vi "OutputWrapper.vi"(0 "VI in":refnum<vi>, 1 "pass":bool, 2 "FinalCluster":T1) -> (3 "PASS":bool, 4 "error out":errorcluster, 5 "ats json out":string, 6 "formatted test json out":string)   [LabVIEW 2019]
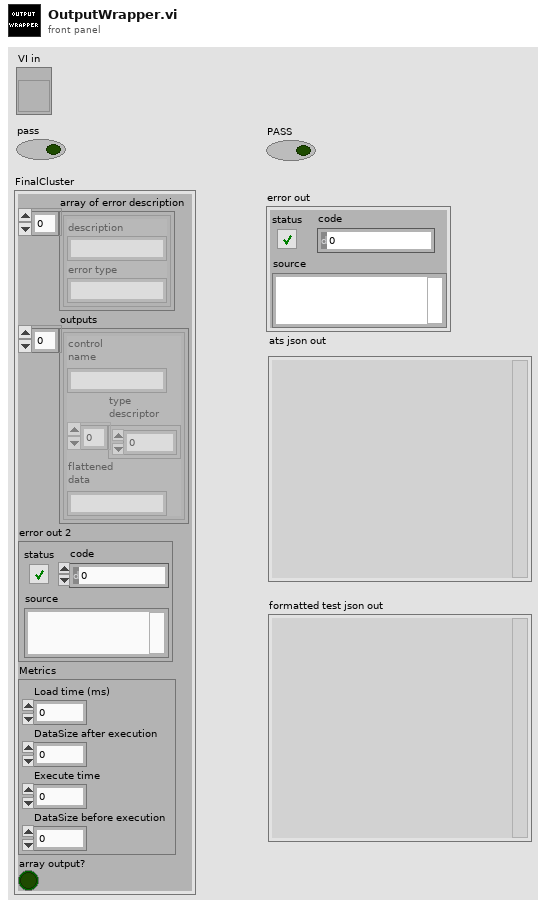
[diagram p1: front panel]
types:
  T1 = cluster{"array of error description":cluster{"description":string, "error type":string}[], "outputs":cluster{"control\nname":string, "type\ndescriptor":i16[], "flattened\ndata":string}[], "error out 2":errorcluster, "Metrics":cluster{"Load time (ms)":u32, "DataSize after execution":u32, "Execute time":u32, "DataSize before execution":u32}, "array output?":bool}
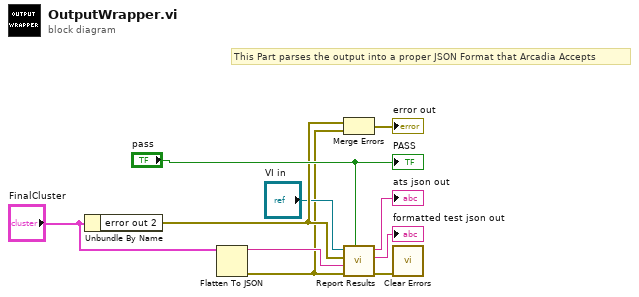
[diagram p0: block diagram]
diagram:
  # "This Part parses the output into a proper JSON Format that Arcadia Accepts"
  n1 = Unbundle By Name("FinalCluster") -> ("error out 2"=w9:errorcluster)
  n2 = Flatten To JSON(anything="FinalCluster") -> (JSON string=w6:string, 11:w3:errorcluster)  [unwired: 2 in]
  n3 = Merge Errors(w9, w3) -> (→"error out":errorcluster)
  n4 = call "Report Results.vi"("pass in"="pass", "error in"=w3, "unformatted test json out"=w6, "test error in"=w9, "vi ref in"="VI in") -> ("error out"=w1:errorcluster, "formatted test json out"=→"formatted test json out":string, "ats json out"=→"ats json out":string)  [unwired: 4 in]
  n5 = call <vilib>:"Clear Errors.vi"("error in (no error)"=w1) -> ()  [unwired: 5 in, 2 out]
  "PASS" <- "pass"
